vi "trueFrameRate.get.vi"(8 "error in (no error)":errorcluster, 11 "trueFrameRate in":refnum<class "trueFrameRate.lvclass">) -> (0 "error out":errorcluster, 2 "trueFrameRate":dbl, 3 "trueFrameRate out":refnum<class "trueFrameRate.lvclass">)   [LabVIEW 2020, in "nominal types.lvlib" / "timestampManifest.lvlib" / "trueFrameRate.lvclass"]
uses:
  trueFrameRate.lvclass
  trueFrameRate.lvclass/trueFrameRate.ctl
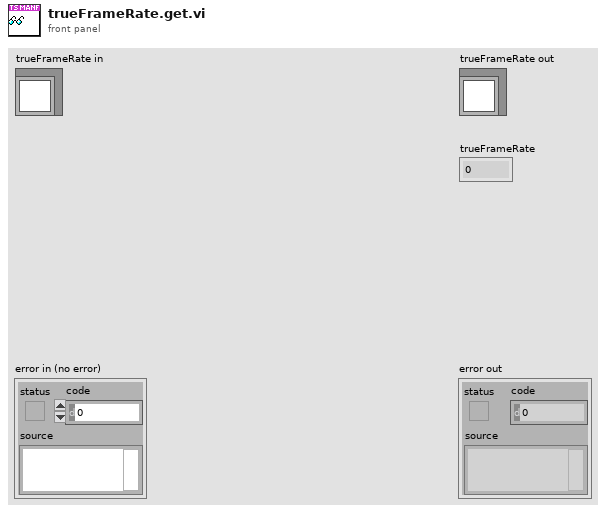
[diagram p1: front panel]
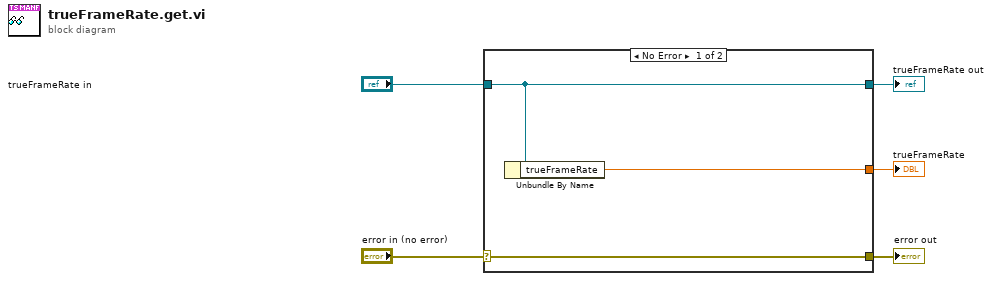
[diagram p0: block diagram]
diagram:
  n1 = case shown="No Error" "error in (no error)" {
    selector: "error in (no error)" -> [w8 w9]
    tunnel: [w8 w9] -> w4
    tunnel: [w7 w10] -> w2
    tunnel: "trueFrameRate in" -> [w7 w10]
    tunnel: [w6 _] -> w1
    frame No Error {
      n2 = Unbundle By Name(w7) -> ("trueFrameRate"=w6:dbl)
    }
    frame Error {
    }
  }
  "error out" <- w4
  "trueFrameRate out" <- w2
  "trueFrameRate" <- w1
